vi "parseReadDACResponse.vi"(8 "error in (no error)":errorcluster, 10 "DynamicFrameParser":refnum<class "DynamicFrameParser.lvclass">, 11 "ILC in":refnum<class "ILC.lvclass">) -> (0 "error out":errorcluster, 3 "ILC out":refnum<class "ILC.lvclass">)   [LabVIEW 2015, in "RTILC.lvlib" / "ILC.lvclass"]
uses:
  ILC.lvclass
  Common_RT_Modbus/DynamicFrameParser/DynamicFrameParser.lvclass
  Common_RT_Modbus/DataTypes/ExceptionCodes.ctl
  ILC.lvclass/ILC.ctl
  Common_RT_Modbus/RTModbus.lvlib
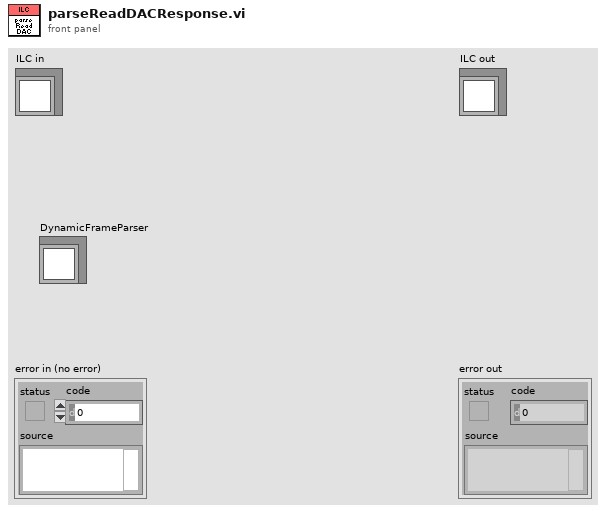
[diagram p1: front panel]
types:
  T1 = typedef "RTModbus.lvlib/ExceptionCodes.ctl" = u16
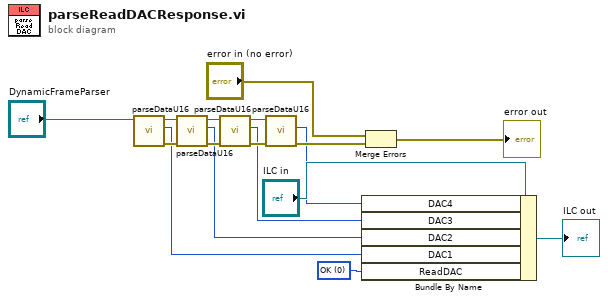
[diagram p0: block diagram]
diagram:
  w15 = T1 0 items=["OK", "IllegalFunction", "IllegalDataAddress", "IllegalDataValue", "SlaveDeviceFailure", "Acknowledge", "SlaveDeviceBusy", "NegativeAcknowledge", "MemoryParityError", "GatewayPathUnavailable", "GatewayTargetDeviceFailedToRespond"] ("ILCData.Responses.ILCMode")
  n1 = call "parseDataU16.vi"("FrameParser in"="DynamicFrameParser") -> ("error out"=w10:errorcluster, "Data"=w4:u16, "FrameParser out"=w13:refnum<class "DynamicFrameParser.lvclass">)  [unwired: 8 in]
  n2 = call "parseDataU16.vi"("error in (no error)"=w10, "FrameParser in"=w13) -> ("error out"=w9:errorcluster, "Data"=w3:u16, "FrameParser out"=w12:refnum<class "DynamicFrameParser.lvclass">)  [unwired: 7 in]
  n3 = call "parseDataU16.vi"("error in (no error)"=w9, "FrameParser in"=w12) -> ("error out"=w8:errorcluster, "Data"=w2:u16, "FrameParser out"=w11:refnum<class "DynamicFrameParser.lvclass">)  [unwired: 7 in]
  n4 = call "parseDataU16.vi"("error in (no error)"=w8, "FrameParser in"=w11) -> ("error out"=w5:errorcluster, "Data"=w1:u16)  [unwired: 7 in, 1 out]
  n5 = Bundle By Name(cluster="ILC in", "DAC4"=w1, "DAC3"=w2, "DAC2"=w3, "DAC1"=w4, "ReadDAC"=w15) -> (→"ILC out":refnum<class "ILC.lvclass">)
  n6 = Merge Errors("error in (no error)", w5) -> (→"error out":errorcluster)
